vi "UpdateWavespec.vi"(8 "error in":errorcluster, 10 "Cluster":T1, 11 "Waveform Specification in":T2) -> (0 "error out":errorcluster, 3 "Waveform Specification out":T2)   [LabVIEW 2017, in "WaveformGenerator.lvlib"]
uses:
  WaveformGenerator.lvlib
  WaveformSpecs.ctl
  WaveformGeneratorInterfaceRef.ctl
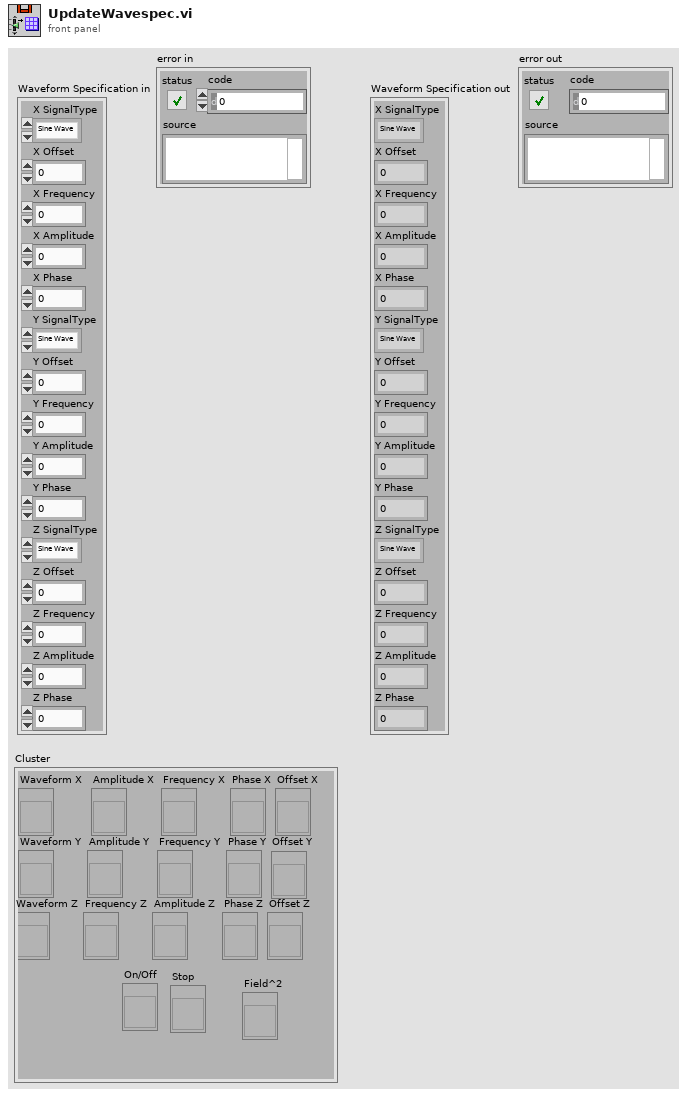
[diagram p1: front panel]
types:
  T1 = typedef "WaveformGenerator.lvlib/WaveformGeneratorInterfaceRef.ctl" = cluster{"Waveform X":refnum<vi>, "Waveform Y":refnum<vi>, "Waveform Z":refnum<vi>, "Amplitude X":refnum<vi>, "Amplitude Y":refnum<vi>, "Amplitude Z":refnum<vi>, "Frequency X":refnum<vi>, "Frequency Y":refnum<vi>, "Frequency Z":refnum<vi>, "Phase X":refnum<vi>, "Phase Y":refnum<vi>, "Phase Z":refnum<vi>, "Offset X":refnum<vi>, "Offset Y":refnum<vi>, "Offset Z":refnum<vi>, "Stop":refnum<vi>, "On/Off":refnum<vi>, "Field^2":refnum<vi>}
  T2 = typedef "WaveformGenerator.lvlib/WaveformSpecs.ctl" = cluster{"X SignalType":enum16{"Sine Wave", "Triangle Wave", "Square Wave", "Sawtooth Wave"}, "X Offset":dbl, "X Frequency":dbl, "X Amplitude":dbl, "X Phase":dbl, "Y SignalType":enum16{"Sine Wave", "Triangle Wave", "Square Wave", "Sawtooth Wave"}, "Y Offset":dbl, "Y Frequency":dbl, "Y Amplitude":dbl, "Y Phase":dbl, "Z SignalType":enum16{"Sine Wave", "Triangle Wave", "Square Wave", "Sawtooth Wave"}, "Z Offset":dbl, "Z Frequency":dbl, "Z Amplitude":dbl, "Z Phase":dbl}
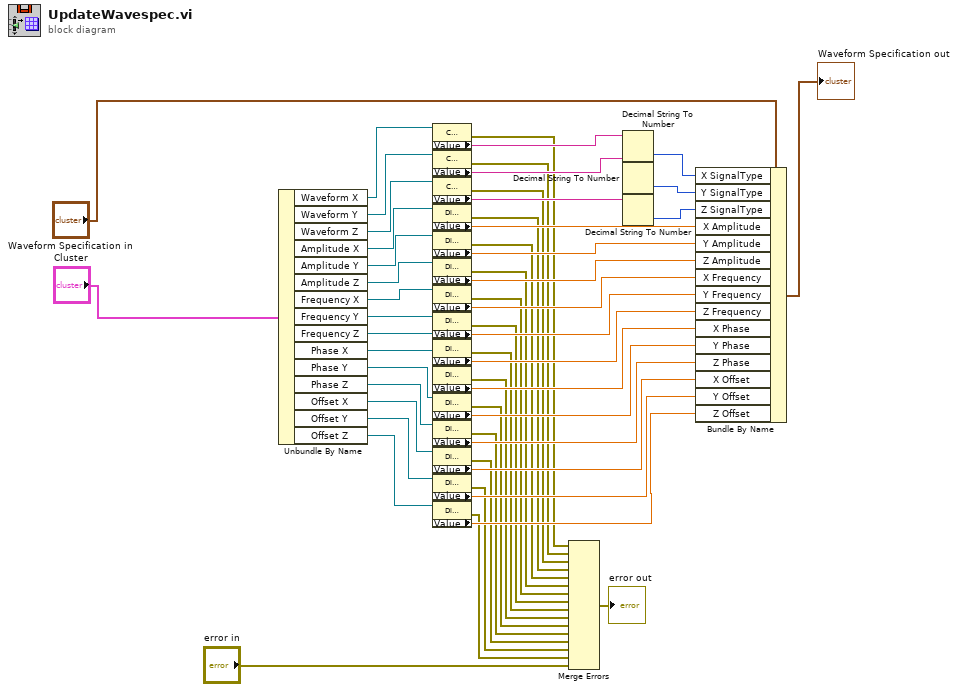
[diagram p0: block diagram]
diagram:
  n1 = Unbundle By Name("Cluster") -> ("Waveform X"=w19:refnum<vi>, "Waveform Y"=w20:refnum<vi>, "Waveform Z"=w21:refnum<vi>, "Amplitude X"=w22:refnum<vi>, "Amplitude Y"=w23:refnum<vi>, "Amplitude Z"=w24:refnum<vi>, "Frequency X"=w25:refnum<vi>, "Frequency Y"=w26:refnum<vi>, "Frequency Z"=w27:refnum<vi>, "Phase X"=w28:refnum<vi>, "Phase Y"=w29:refnum<vi>, "Phase Z"=w33:refnum<vi>, "Offset X"=w30:refnum<vi>, "Offset Y"=w31:refnum<vi>, "Offset Z"=w32:refnum<vi>)
  n2 = property class="CmbBox"(reference=w19) -> (error out=w3:errorcluster, "Value"=w34:string)  [unwired: 1 in, 1 out]
  n3 = property class="CmbBox"(reference=w20) -> (error out=w4:errorcluster, "Value"=w35:string)  [unwired: 1 in, 1 out]
  n4 = property class="CmbBox"(reference=w21) -> (error out=w5:errorcluster, "Value"=w52:string)  [unwired: 1 in, 1 out]
  n5 = property class="DigNum (strict)"(reference=w22) -> (error out=w6:errorcluster, "Value"=w39:dbl)  [unwired: 1 in, 1 out]
  n6 = property class="DigNum (strict)"(reference=w23) -> (error out=w7:errorcluster, "Value"=w40:dbl)  [unwired: 1 in, 1 out]
  n7 = property class="DigNum (strict)"(reference=w24) -> (error out=w8:errorcluster, "Value"=w41:dbl)  [unwired: 1 in, 1 out]
  n8 = property class="DigNum (strict)"(reference=w25) -> (error out=w9:errorcluster, "Value"=w42:dbl)  [unwired: 1 in, 1 out]
  n9 = property class="DigNum (strict)"(reference=w26) -> (error out=w10:errorcluster, "Value"=w43:dbl)  [unwired: 1 in, 1 out]
  n10 = property class="DigNum (strict)"(reference=w27) -> (error out=w11:errorcluster, "Value"=w44:dbl)  [unwired: 1 in, 1 out]
  n11 = property class="DigNum (strict)"(reference=w28) -> (error out=w12:errorcluster, "Value"=w45:dbl)  [unwired: 1 in, 1 out]
  n12 = property class="DigNum (strict)"(reference=w29) -> (error out=w13:errorcluster, "Value"=w46:dbl)  [unwired: 1 in, 1 out]
  n13 = property class="DigNum (strict)"(reference=w33) -> (error out=w14:errorcluster, "Value"=w47:dbl)  [unwired: 1 in, 1 out]
  n14 = property class="DigNum (strict)"(reference=w30) -> (error out=w15:errorcluster, "Value"=w48:dbl)  [unwired: 1 in, 1 out]
  n15 = property class="DigNum (strict)"(reference=w31) -> (error out=w16:errorcluster, "Value"=w49:dbl)  [unwired: 1 in, 1 out]
  n16 = property class="DigNum (strict)"(reference=w32) -> (error out=w17:errorcluster, "Value"=w50:dbl)  [unwired: 1 in, 1 out]
  n17 = Merge Errors(w3, w4, w5, w6, w7, w8, w9, w10, w11, w12, w13, w14, w15, w16, w17, "error in") -> (→"error out":errorcluster)
  n18 = Decimal String To Number(string=w34) -> (number=w36:i32)  [unwired: 2 in, 1 out]
  n19 = Decimal String To Number(string=w35) -> (number=w37:i32)  [unwired: 2 in, 1 out]
  n20 = Decimal String To Number(string=w52) -> (number=w38:i32)  [unwired: 2 in, 1 out]
  n21 = Bundle By Name(cluster="Waveform Specification in", "X SignalType"=w36, "Y SignalType"=w37, "Z SignalType"=w38, "X Amplitude"=w39, "Y Amplitude"=w40, "Z Amplitude"=w41, "X Frequency"=w42, "Y Frequency"=w43, "Z Frequency"=w44, "X Phase"=w45, "Y Phase"=w46, "Z Phase"=w47, "X Offset"=w48, "Y Offset"=w49, "Z Offset"=w50) -> (→"Waveform Specification out":T2)
